vi "circuito.vi"() -> ()   [LabVIEW 2019]
panel:
  out "Potencia":dbl format="%#_4g"
  out "Voltios  R":dbl format="%#_4g"
  in  "Resistencia 1":dbl(slide) scale=0.0..10.0
  in  "Resistencia 2":dbl(slide) scale=0.0..10.0
  in  "Voltios":dbl(slide) scale=0.0..10.0
  out "Amperimetro":dbl(knob) scale=0.0..10.0
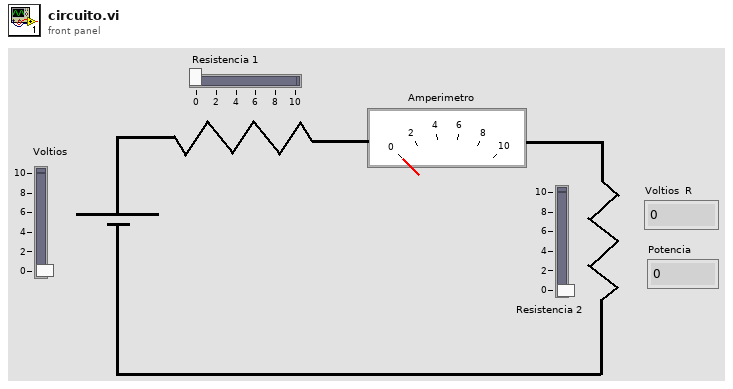
[diagram p1: front panel]
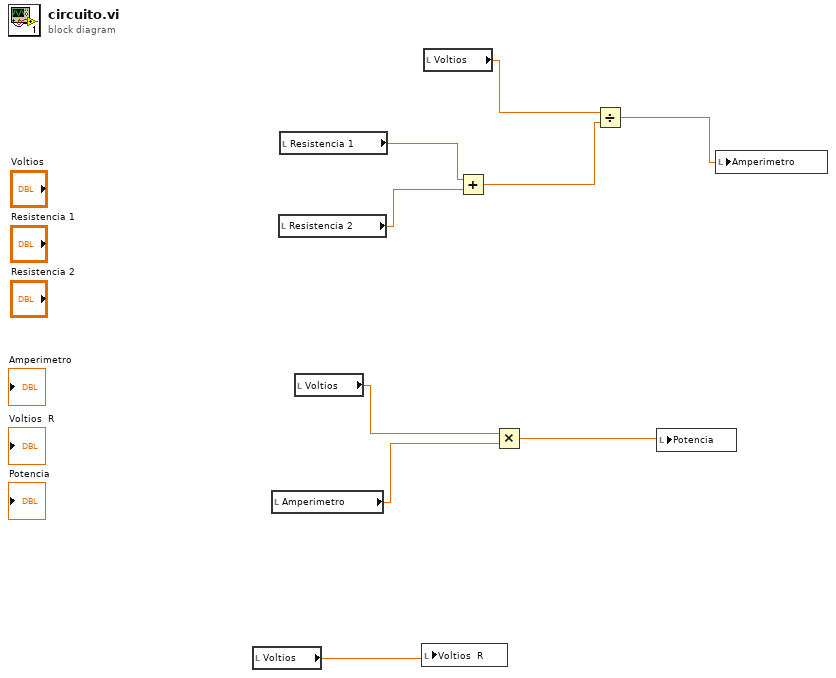
[diagram p0: block diagram]
diagram:
  n1 = local read "Voltios"() -> (w1:dbl)
  n2 = local read "Amperimetro"() -> (w9:dbl)
  n3 = local read "Resistencia 2"() -> (w6:dbl)
  n4 = local read "Resistencia 1"() -> (w5:dbl)
  n5 = local read "Voltios"() -> (w8:dbl)
  n6 = local write "Voltios  R"(w1) -> ()
  n7 = local read "Voltios"() -> (w4:dbl)
  n8 = Add(x=w5, y=w6) -> (x+y=w3:dbl)
  n9 = Multiply(x=w8, y=w9) -> (x*y=w7:dbl)
  n10 = Divide(x=w4, y=w3) -> (x/y=w2:dbl)
  n11 = local write "Potencia"(w7) -> ()
  n12 = local write "Amperimetro"(w2) -> ()
